vi "encoder_sub.vi"(0 "A_pre":bool, 1 "B_pre":bool, 3 "Encoder Position_pre":i32, 10 "A input":bool, 11 "Encoder Position Reset":bool, 14 "B input":bool) -> (20 "A":bool, 21 "B":bool, 23 "Encoder Position (Counts)":i32)   [LabVIEW 2014]
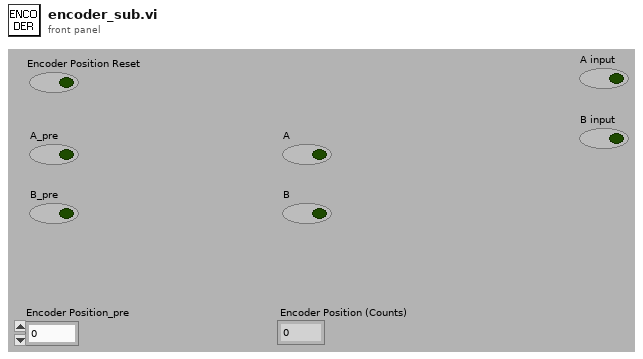
[diagram p1: front panel]
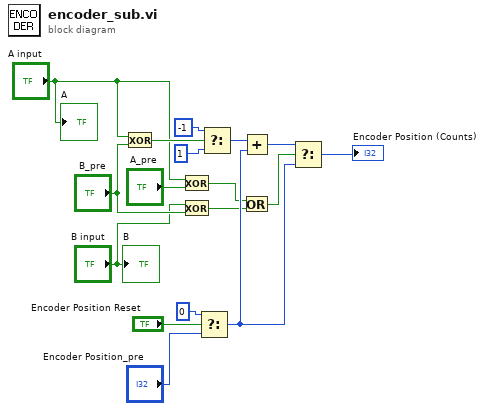
[diagram p0: block diagram]
diagram:
  n1 = Exclusive Or(1:"B_pre", 2:"A input") -> (0:w9:bool)
  n2 = Exclusive Or(1:"A_pre", 2:"A input") -> (0:w10:bool)
  n3 = Exclusive Or(1:"B_pre", 2:"B input") -> (0:w11:bool)
  n4 = Select(t=0 ("32 bit"), s="Encoder Position Reset", f="Encoder Position_pre") -> (s? t:f=w15:i32)
  n5 = Select(t=-1 ("32 bit"), s=w9, f=1 ("32 bit")) -> (s? t:f=w14:i32)
  n6 = Add(x=w14, y=w15) -> (x+y=w17:i32)
  n7 = Or(x=w10, y=w11) -> (x .or. y?=w8:bool)
  n8 = Select(t=w17, s=w8, f=w15) -> (s? t:f=→"Encoder Position (Counts)":i32)
  "A" <- "A input"
  "B" <- "B input"
